vi "BatteryToString.vi"(8 "error in (no error)":errorcluster, 11 "Battery":dbl) -> (0 "error out":errorcluster, 3 "Battery String":string)   [LabVIEW 2012]
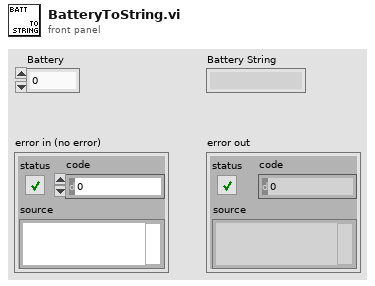
[diagram p1: front panel]
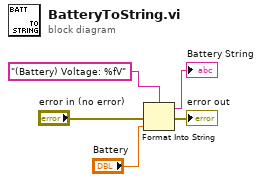
[diagram p0: block diagram]
diagram:
  n1 = Format Into String(format string="(Battery) Voltage: %fV", error in="error in (no error)", "Battery") -> (resulting string=→"Battery String":string, error out=→"error out":errorcluster)  [unwired: 1 in]
